vi "test ai read.vi"() -> ()   [LabVIEW 2012]
uses:
  <vilib>/rvi/eio/common/nirviEmuTemplateMethod_errors.vi
  <vilib>/eio/EIONode/EIONode.xnode
panel:
  out "Connector0/AI7":i16
  out "Connector0/AI6":i16
  out "Connector0/AI5":i16
  out "Connector0/AI4":i16
  out "Connector0/AI3":i16
  out "Connector0/AI2":i16
  out "Connector0/AI1":i16
  out "Connector0/AI0":i16
  in  "ai count":u32=4000
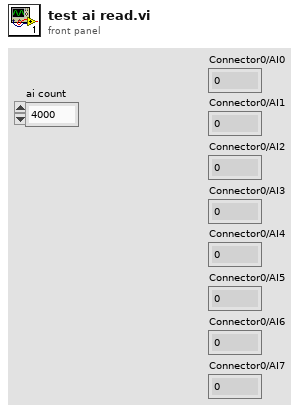
[diagram p1: front panel]
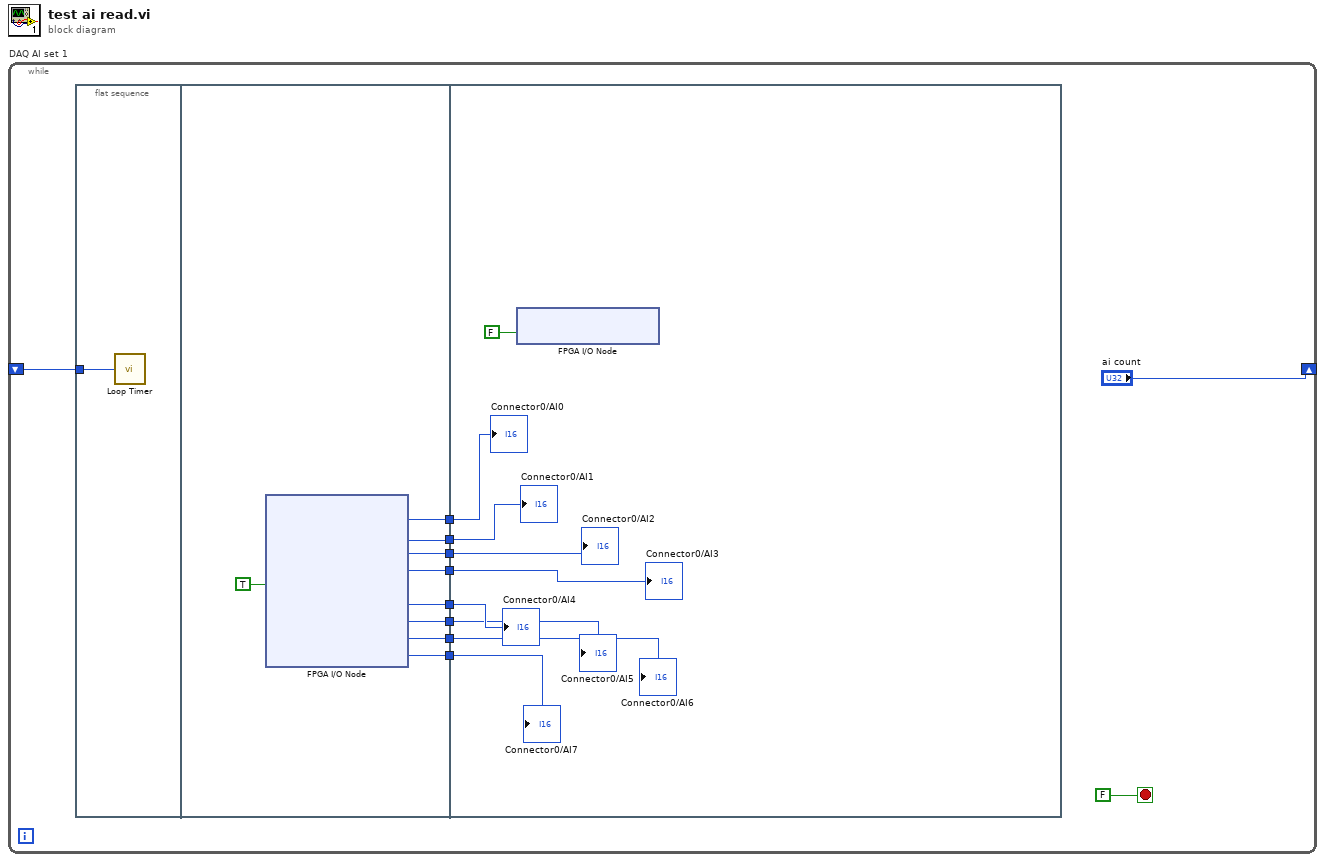
[diagram p0: block diagram]
diagram:
  n1 = while "DAQ AI set 1" {
    shift-right: ["ai count"] -> _
    shift-left: _ -> [w2]
    stop <- FALSE stop-if-true
    n2 = flat-sequence {
      tunnel: w2 -> [w12]
      tunnel: [w20] -> w10
      tunnel: [w19] -> w9
      tunnel: [w18] -> w8
      tunnel: [w17] -> w7
      tunnel: [w16] -> w6
      tunnel: [w15] -> w5
      tunnel: [w14] -> w4
      tunnel: [w13] -> w3
      tunnel: w10 -> [w29]
      tunnel: w9 -> [w28]
      tunnel: w8 -> [w27]
      tunnel: w7 -> [w26]
      tunnel: w6 -> [w25]
      tunnel: w5 -> [w24]
      tunnel: w4 -> [w23]
      tunnel: w3 -> [w22]
      frame #0 {
        n3 = call "Loop Timer"("Count(Ticks)"=w12) -> ()  [unwired: 1 out]
      }
      frame #1 {
        n4 = xnode "FPGA I/O Node"("Connector1/DIO31"=TRUE ("Connector1/DIO33")) -> ("Connector0/AI0"=w20:i16, "Connector0/AI1"=w19:i16, "Connector0/AI2"=w18:i16, "Connector0/AI3"=w17:i16, "Connector0/AI4"=w16:i16, "Connector0/AI5"=w15:i16, "Connector0/AI6"=w14:i16, "Connector0/AI7"=w13:i16)  [unwired: 9 in, 9 out]
      }
      frame #2 {
        n5 = xnode "FPGA I/O Node"("Connector1/DIO31"=FALSE ("Connector1/DIO34")) -> ()  [unwired: 1 in, 1 out]
        "Connector0/AI0" <- w29
        "Connector0/AI1" <- w28
        "Connector0/AI2" <- w27
        "Connector0/AI3" <- w26
        "Connector0/AI4" <- w25
        "Connector0/AI5" <- w24
        "Connector0/AI6" <- w23
        "Connector0/AI7" <- w22
      }
    }
  }
